vi "New Panel Selected.vi"(8 "error in (no error)":errorcluster, 10 "Chat Window":i32(listbox), 11 "SubPanel User Interface in":refnum<class "SubPanel User Interface.lvclass">) -> (0 "error out":errorcluster, 3 "SubPanel User Interface out":refnum<class "SubPanel User Interface.lvclass">)   [LabVIEW 2015, in "SubPanel User Interface.lvlib" / "SubPanel User Interface.lvclass"]
uses:
  SubPanel User Interface.lvclass
  SubPanel User Interface.lvclass/SubPanel User Interface.ctl
  UI Reference Wrapper/UI Reference Wrapper.lvclass
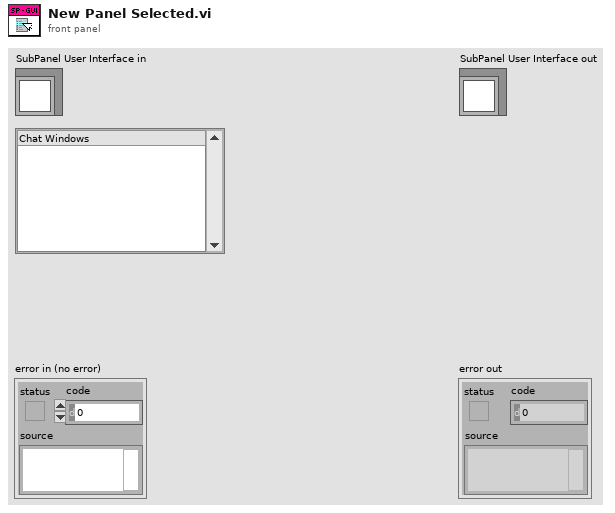
[diagram p1: front panel]
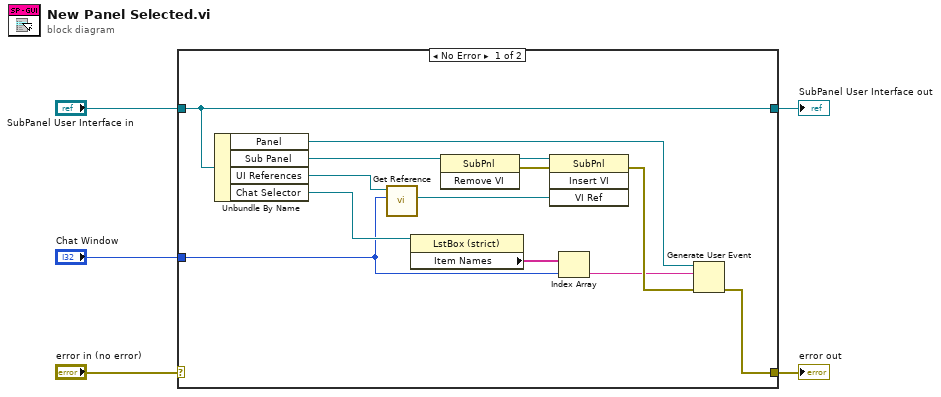
[diagram p0: block diagram]
diagram:
  n1 = case shown="No Error" "error in (no error)" {
    selector: "error in (no error)" -> [_ w20]
    tunnel: [w12 w20] -> w4
    tunnel: [w18 w19] -> w2
    tunnel: "SubPanel User Interface in" -> [w18 w19]
    tunnel: "Chat Window" -> [w7 _]
    frame No Error {
      n2 = Unbundle By Name(w18) -> ("Panel"=w14:refnum<user-event>, "Sub Panel"=w15:refnum<vi>, "UI References"=w8:refnum<class "UI Reference Wrapper.lvclass">, "Chat Selector"=w11:refnum<vi>)
      n3 = call "Get Reference.vi"("Numeric"=w7, "UI Reference Wrapper in"=w8) -> ("VI Refnum"=w6:refnum<vi>)  [unwired: 6 in, 3 out]
      n4 = property class="LstBox (strict)"(reference=w11) -> ("Item Names"=w10:string[])  [unwired: 1 in, 2 out]
      n5 = invoke class="SubPnl" method="Remove VI"(reference=w15) -> (reference out=w17:refnum<vi>, error out=w16:errorcluster)  [unwired: 2 in, 1 out]
      n6 = invoke class="SubPnl" method="Insert VI"(reference=w17, error in=w16, "VI Ref"=w6) -> (error out=w13:errorcluster)  [unwired: 1 in, 3 out]
      n7 = Index Array(array=w10, index=w7) -> (element=w9:string)
      n8 = Generate User Event(user event=w14, event data cluster=w9, error in=w13) -> (error out=w12:errorcluster)  [unwired: 1 in, 1 out]
    }
    frame Error {
    }
  }
  "error out" <- w4
  "SubPanel User Interface out" <- w2
